vi "adding a sine signal.vi"() -> ()   [LabVIEW 2017]
uses:
  <vilib>/measure/NI_MABase.lvlib
panel:
  out "sine signal":waveform(dbl)(graph)
  out "main signal":waveform(dbl)[](graph)
  out "x+y":waveform(dbl)[](graph)
  out "x+y":waveform(dbl)[](array[waveform])
  in  "path 3":path
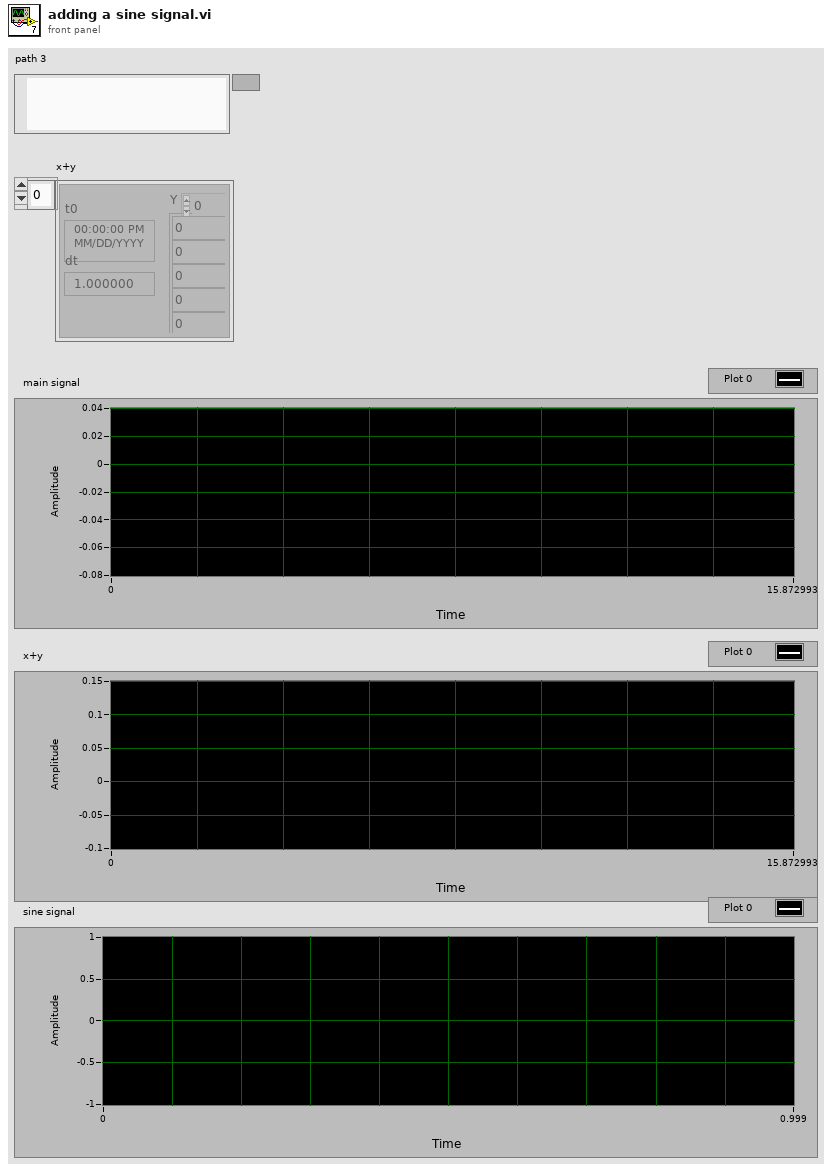
[diagram p1: front panel]
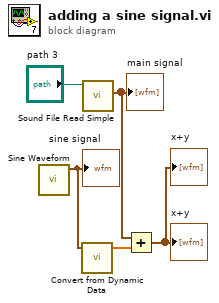
[diagram p0: block diagram]
diagram:
  n1 = call <vilib>:"Sine Waveform.vi"() -> ("signal out"=w1:waveform(dbl))  [unwired: 10 in, 1 out]
  "sine signal" <- w1
  n2 = call "Convert from Dynamic Data"("Dynamic Data Type"=w1) -> ("Array"=w2:dbl[])  [unwired: 3 in]
  n3 = call <vilib>:"Sound File Read Simple.vi"("path"="path 3") -> ("data"=w3:waveform(dbl)[])  [unwired: 7 in, 3 out]
  "main signal" <- w3
  n4 = Add(x=w3, y=w2) -> (x+y=→"x+y" →"x+y":waveform(dbl)[])
